vi "3Tab切換.vi"() -> ()   [LabVIEW 2019]
panel:
  in  "Stop":bool
  in  "下一步":bool
  in  "上一步":bool
  in  "請購流程":enum32{"建立請購清單", "金額計算", "付款"}(tab)
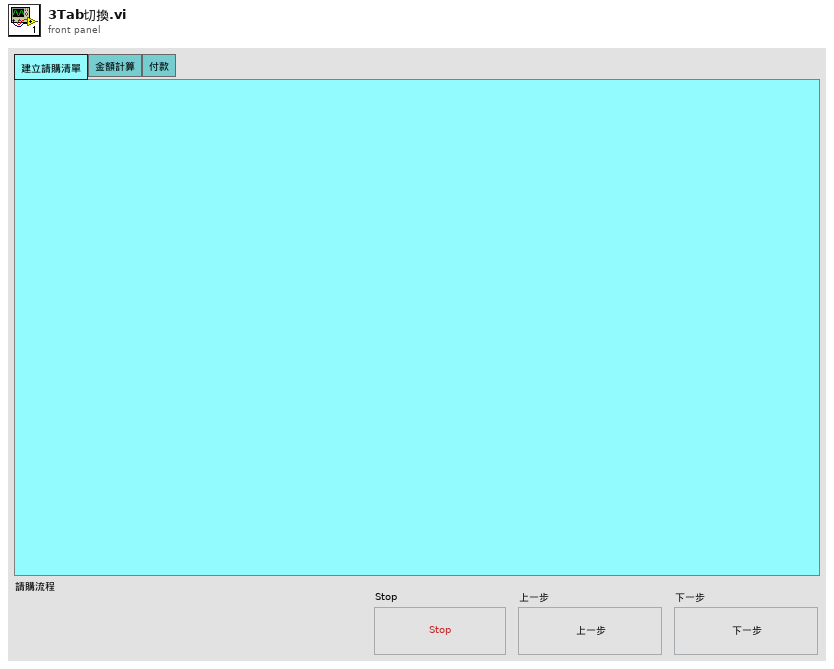
[diagram p1: front panel]
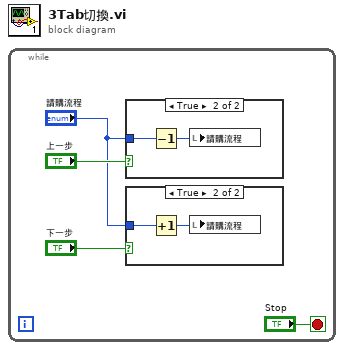
[diagram p0: block diagram]
diagram:
  n1 = while {
    stop <- "Stop" stop-if-true
    n2 = case shown="True" "上一步" {
      tunnel: "請購流程" -> [_ w8]
      frame False {
      }
      frame True {
        n3 = Decrement(x=w8) -> (x-1=w7:enum32{"建立請購清單", "金額計算", "付款"})
        n4 = local write "請購流程"(w7) -> ()
      }
    }
    n5 = case shown="True" "下一步" {
      tunnel: "請購流程" -> [_ w6]
      frame False {
      }
      frame True {
        n6 = Increment(x=w6) -> (x+1=w5:enum32{"建立請購清單", "金額計算", "付款"})
        n7 = local write "請購流程"(w5) -> ()
      }
    }
  }
